vi "bigboytest.vi"() -> ()   [LabVIEW 2012, in "MainProject.lvrbt"]
uses:
  MainProject.lvrbt
  Drivers/AutoDriverControl.ctl
  <vilib>/NXT/Hardware/Plugins/Tetrix DC Motor/TetrixDCMotorAddress.ctl
  <vilib>/NXT/HiTechnic/HiTechnic Controls/HiTechnic Port.ctl
  <vilib>/NXT/Block Support/NXT_InputPort.ctl
  <vilib>/NXT/Dual Mode Library/Sound/Tone.vi
  <vilib>/NXT/NXTIO Xnodes/AddressXNode/NXTIOAddress.xnode
panel:
  out "Color":string="Black"
  in  "stop":bool
  out "Detected Line?":bool
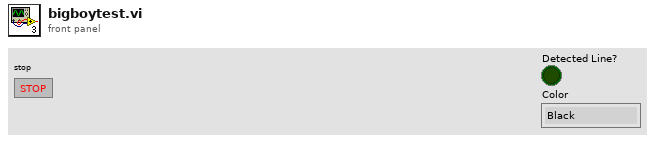
[diagram p1: front panel]
types:
  T1 = typedef "AutoDriverControl.ctl" = enum16{"Init", "Forward", "Reverse", "Left", "Right", "Brake"}
  T2 = typedef "TetrixDCMotorAddress.ctl" = i16
  T3 = typedef "LVHSConnector.ctl" = refnum<class "BrickReference.lvclass">
  T4 = typedef "HiTechnic Port.ctl" = cluster{"Port":T5, "MUX Port":u8}
  T5 = typedef "NXT_InputPort.ctl" = u8
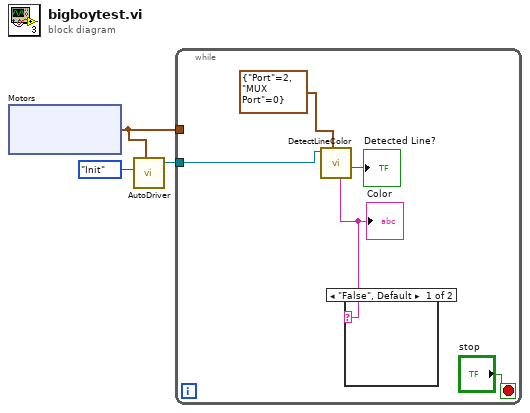
[diagram p0: block diagram]
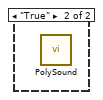
[diagram p2: hidden frame]
diagram:
  n1 = xnode "Motors"() -> ("Motor"=w3:cluster{"TetrixDCMotor":T2, "TetrixDCMotor":T2})
  n2 = call "AutoDriver.vi"("Motors"=w3, "Direction"=AutoDriverControl."Init") -> ("NXT Out"=w2:T3)  [unwired: 6 in]
  n3 = while {
    tunnel: w3 -> [_]
    tunnel: w2 -> [w4]
    stop <- "stop" stop-if-true
    n4 = call "DetectLineColor.vi"("Port/MUX"=T4 {"Port"=2, "MUX Port"=0}, "NXT In"=w4) -> ("Detected Line?"=→"Detected Line?":bool, "Color"=w6:string)  [unwired: 7 in, 1 out]
    "Color" <- w6
    n5 = case shown="\"False\", Default" w6 {
      frame "False", Default {
      }
      frame "True" {
        n6 = call-poly <vilib>:"PolySound.vi"() -> ()  [unwired: 4 in, 1 out]
      }
    }
  }
